vi "Header.CreateRequests.vi"(8 "error in (no error)":errorcluster) -> (0 "error out":errorcluster, 3 "Requests":T1)   [LabVIEW 2024, in "Header.lvclass"]
uses:
  Header.lvclass
  Request Events--cluster.ctl
  Do Something Args.ctl
  RQMHCore/ModuleCore/Reply.ctl
  Add Menu Item Args.ctl
  Header.lvclass/Header.ctl
  RQMHCore/ModuleCore/RQMHModule.lvclass
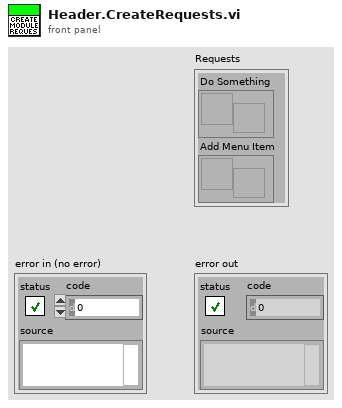
[diagram p1: front panel]
types:
  T1 = typedef "Header.lvclass/Request Events--cluster.ctl" = cluster{"Do Something":refnum<user-event>, "Add Menu Item":refnum<user-event>}
  T2 = typedef "Header.lvclass/Add Menu Item Args.ctl" = cluster{"Item":string}
  T3 = typedef "RQMHModule.lvclass/Reply.ctl" = cluster{"Expects Reply":bool, "Reply":refnum<notifier>}
  T4 = typedef "Header.lvclass/Do Something Args.ctl" = cluster{"Msg":string}
  T5 = cluster{"Do Something Args":T4, "Reply Payload":T3}
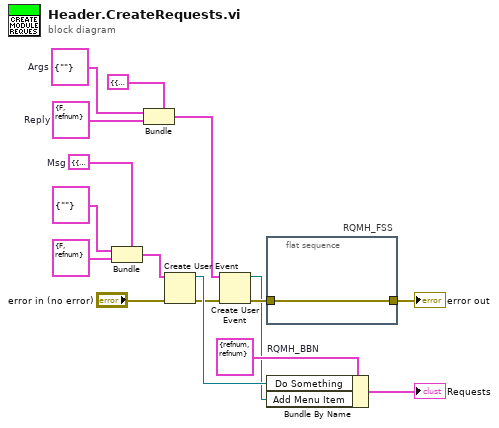
[diagram p0: block diagram]
diagram:
  w4 = T2 {"Item"=""}  # Args
  w3 = T3 {"Expects Reply"=FALSE, "Reply"=refnum}  # Reply
  w10 = T5 {"Do Something Args"={"Msg"=""}, "Reply Payload"={"Expects Reply"=FALSE, "Reply"=refnum}}  # Msg
  n1 = Bundle(cluster=w10, "Do Something Args"=T4 {"Msg"=""}, "Reply Payload"=T3 {"Expects Reply"=FALSE, "Reply"=refnum}) -> (w13:T5)
  n2 = Bundle(cluster=cluster{"Args":T2, "Reply":T3} {"Args"={"Item"=""}, "Reply"={"Expects Reply"=FALSE, "Reply"=refnum}} ("Msg"), "Args"=w4, "Reply"=w3) -> (w2:cluster{"Args":T2, "Reply":T3})
  n3 = Create User Event(user event datatype=w13, error in="error in (no error)") -> (user event=w9:refnum<user-event>, error out=w7:errorcluster)
  n4 = Create User Event(user event datatype=w2, error in=w7) -> (user event=w5:refnum<user-event>, error out=w6:errorcluster)
  n5 = flat-sequence "RQMH_FSS" {
    tunnel: [w17] -> w8
    tunnel: w6 -> [w17]
    frame #0 {
    }
  }
  n6 = Bundle By Name "RQMH_BBN"(cluster=T1 {"Do Something"=refnum, "Add Menu Item"=refnum} ("Requests"), "Do Something"=w9, "Add Menu Item"=w5) -> (→"Requests":T1)
  "error out" <- w8
